vi "Rx.vi"(8 "error in (no error)":errorcluster, 10 "Transfer Group in":refnum<class "Transfer Group.lvclass">, 11 "Transceiver Thread in":refnum<class "Transceiver Thread.lvclass">) -> (0 "error out":errorcluster, 2 "Transfer Group out":refnum<class "Transfer Group.lvclass">, 3 "Transceiver Thread out":refnum<class "Transceiver Thread.lvclass">)   [LabVIEW 2021, in "DSF Core.lvlib" / "Transceiver Thread.lvclass"]
uses:
  Transceiver Thread.lvclass
  Transfer Group/Transfer Group.lvclass
  Transceiver Thread.lvclass/Transceiver Thread.ctl
  Transfer Group/Transfer Group.lvclass/Transfer Group.ctl
  Transceiver/Transceiver.lvclass
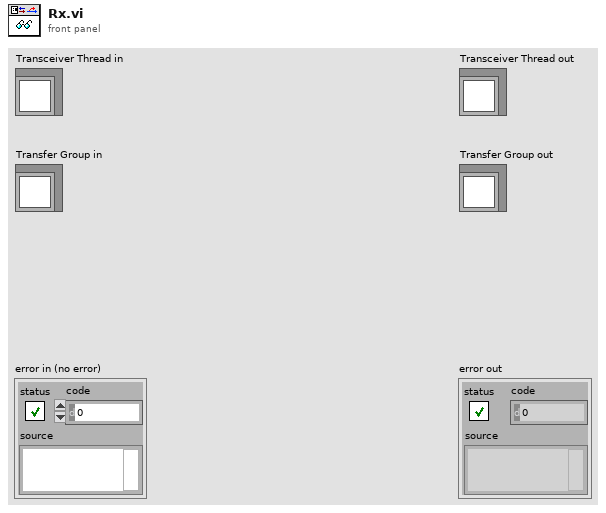
[diagram p1: front panel]
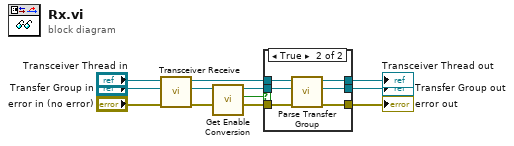
[diagram p0: block diagram]
diagram:
  n1 = call "Transceiver Receive.vi"("error in (no error)"="error in (no error)", "Transfer Group in"="Transfer Group in", "Transceiver Thread in"="Transceiver Thread in") -> ("error out"=w11:errorcluster, "Transfer Group out"=w3:refnum<class "Transfer Group.lvclass">, "Transceiver Thread out"=w4:refnum<class "Transceiver Thread.lvclass">)  [unwired: 6 in]
  n2 = call "Get Enable Conversion.vi"("Transfer Group in"=w3) -> ("enable conversion"=w1:bool, "Transfer Group out"=w2:refnum<class "Transfer Group.lvclass">)  [unwired: 9 in]
  n3 = case shown="True" w1 {
    tunnel: w11 -> [w14 w20]
    tunnel: [w13 w19] -> w9
    tunnel: [w14 w18] -> w6
    tunnel: [w12 w17] -> w5
    tunnel: w4 -> [w13 w16]
    tunnel: w2 -> [w12 w15]
    frame False {
    }
    frame True {
      n4 = call "Parse Transfer Group.vi"("error in (no error)"=w20, "Transfer Group in"=w15, "Plugin Thread in"=w16) -> ("error out"=w18:errorcluster, "Transfer Group out"=w17:refnum<class "Transfer Group.lvclass">, "Plugin Thread out"=w19:refnum<class "Transceiver Thread.lvclass">)  [unwired: 6 in]
    }
  }
  "error out" <- w6
  "Transceiver Thread out" <- w9
  "Transfer Group out" <- w5
